vi "Encode DCW Parameters - 24ch.vi"(8 "ADD Parameters (in)":string, 9 "Scanner Settings":T2={"Scan1"=1, "Scan2"=1, "Scan3"=1, "Scan4"=1, "Scan5"=1, "Scan6"=1, "Scan7"=1, "Scan8"=1, "Scan9"=1, "Scan10"=1, "Scan11"=1, "Scan12"=1, "Scan13"=1, "Scan14"=1, "Scan15"=1, "Scan16"=1, "Scan17"=1, "Scan10 2"=1, "Scan11 2"=1, "Scan12 2"=1, "Scan13 2"=1, "Scan14 2"=1, "Scan15 2"=1, "Scan24"=1} {"Scan24" scale=0.0..2.0; "Scan15 2" scale=0.0..2.0; "Scan14 2" scale=0.0..2.0; "Scan13 2" scale=0.0..2.0; "Scan12 2" scale=0.0..2.0; "Scan11 2" scale=0.0..2.0; "Scan10 2" scale=0.0..2.0; "Scan17" scale=0.0..2.0; "Scan16" scale=0.0..2.0; "Scan15" scale=0.0..2.0; "Scan14" scale=0.0..2.0; "Scan13" scale=0.0..2.0; "Scan12" scale=0.0..2.0; "Scan11" scale=0.0..2.0; "Scan10" scale=0.0..2.0; "Scan9" scale=0.0..2.0; "Scan8" scale=0.0..2.0; "Scan7" scale=0.0..2.0; "Scan6" scale=0.0..2.0; "Scan5" scale=0.0..2.0; "Scan4" scale=0.0..2.0; "Scan3" min=0 max=2 scale=0.0..2.0; "Scan2" min=0 max=2 scale=0.0..2.0; "Scan1" min=0 max=2 scale=0.0..2.0}, 10 "Internal Scanner Exists?":bool, 11 "DCW Test Parameters out":T1={"Voltage (1500)"=1500, "High Limit(0.0 - 10,000 microamps) (10)"=10000.0, "Low Limit(0.0 - 10,000 microamps) (0)"=0.0, "Ramp Up Time (0.4 - 999.9 seconds) (0.4)"=0.4, "Dwell Time (0, 0.4 - 999.9 seconds) (1)"=1.0, "Ramp Down Time (0, 1.0 - 999.9 seconds) (0) "=0.0, "Charge LO (0.0 - 350uA)"=0.0, "Arc Sense (1 - 9) (5)"=5, "Arc Detect (F: Off)"=FALSE, "Continuity (F: Off)"=FALSE, "Auto Charge LO (F: Off)"=FALSE, "Low Range (F: Off)"=FALSE, "Offset (0.0 - 10,000uA)"=0.0, "Ramp-Hi (0.0 - 10,000uA)"=0.0, "Range (F: AUTO)"=enum."AUTO"} {"Ramp-Hi (0.0 - 10,000uA)" format="%.2f"; "Offset (0.0 - 10,000uA)" format="%.2f"; "Ramp Down Time (0, 1.0 - 999.9 seconds) (0)" format="%.1f"; "Charge LO (0.0 - 350uA)" format="%.2f"; "Dwell Time (0, 0.4 - 999.9 seconds) (1)" format="%.1f"; "Ramp Up Time (0.4 - 999.9 seconds) (0.4)" format="%.1f"; "Low Limit(0.0 - 10,000 microamps) (0)" format="%.1f"; "High Limit(0.0 - 10,000 microamps) (10)" format="%.1f"}) -> (0 "Scanner Settings":T2={"Scan1"=1, "Scan2"=1, "Scan3"=1, "Scan4"=1, "Scan5"=1, "Scan6"=1, "Scan7"=1, "Scan8"=1, "Scan9"=1, "Scan10"=1, "Scan11"=1, "Scan12"=1, "Scan13"=1, "Scan14"=1, "Scan15"=1, "Scan16"=1, "Scan17"=1, "Scan10 2"=1, "Scan11 2"=1, "Scan12 2"=1, "Scan13 2"=1, "Scan14 2"=1, "Scan15 2"=1, "Scan24"=1} {"Scan24" scale=0.0..2.0; "Scan15 2" scale=0.0..2.0; "Scan14 2" scale=0.0..2.0; "Scan13 2" scale=0.0..2.0; "Scan12 2" scale=0.0..2.0; "Scan11 2" scale=0.0..2.0; "Scan10 2" scale=0.0..2.0; "Scan17" scale=0.0..2.0; "Scan16" scale=0.0..2.0; "Scan15" scale=0.0..2.0; "Scan14" scale=0.0..2.0; "Scan13" scale=0.0..2.0; "Scan12" scale=0.0..2.0; "Scan11" scale=0.0..2.0; "Scan10" scale=0.0..2.0; "Scan9" scale=0.0..2.0; "Scan8" scale=0.0..2.0; "Scan7" scale=0.0..2.0; "Scan6" scale=0.0..2.0; "Scan5" scale=0.0..2.0; "Scan4" scale=0.0..2.0; "Scan3" min=0 max=2 scale=0.0..2.0; "Scan2" min=0 max=2 scale=0.0..2.0; "Scan1" min=0 max=2 scale=0.0..2.0}, 1 "DCW Test Parameters out":T1={"Voltage (1500)"=1500, "High Limit(0.0 - 10,000 microamps) (10)"=10000.0, "Low Limit(0.0 - 10,000 microamps) (0)"=0.0, "Ramp Up Time (0.4 - 999.9 seconds) (0.4)"=0.4, "Dwell Time (0, 0.4 - 999.9 seconds) (1)"=1.0, "Ramp Down Time (0, 1.0 - 999.9 seconds) (0) "=0.0, "Charge LO (0.0 - 350uA)"=0.0, "Arc Sense (1 - 9) (5)"=5, "Arc Detect (F: Off)"=FALSE, "Continuity (F: Off)"=FALSE, "Auto Charge LO (F: Off)"=FALSE, "Low Range (F: Off)"=FALSE, "Offset (0.0 - 10,000uA)"=0.0, "Ramp-Hi (0.0 - 10,000uA)"=0.0, "Range (F: AUTO)"=enum."AUTO"} {"Ramp-Hi (0.0 - 10,000uA)" format="%.2f"; "Offset (0.0 - 10,000uA)" format="%.2f"; "Ramp Down Time (0, 1.0 - 999.9 seconds) (0)" format="%.1f"; "Charge LO (0.0 - 350uA)" format="%.2f"; "Dwell Time (0, 0.4 - 999.9 seconds) (1)" format="%.1f"; "Ramp Up Time (0.4 - 999.9 seconds) (0.4)" format="%.1f"; "Low Limit(0.0 - 10,000 microamps) (0)" format="%.1f"; "High Limit(0.0 - 10,000 microamps) (10)" format="%.1f"}, 3 "Add Parameters":string)   [LabVIEW 2020, in "Associated Research 78XX Series.lvlib"]
uses:
  <instrlib>/Associated Research 78XX Series/Associated Research 78XX Series.lvlib
  <instrlib>/Associated Research 78XX Series/Public/Configure/Steps/Low Level/Scanner Settings - 24ch.ctl
  <instrlib>/Associated Research 78XX Series/Public/Configure/Steps/Low Level/DCW Test Parameters.ctl
panel:
  # "On\nOff"
  # "On\nOff"
  # "On\nOff"
  # "Fixed\nAuto"
  # "On\nOff"
  # "On\nOff"
  # "On\nOff"
  # "On\nOff"
  # "Fixed\nAuto"
  # "On\nOff"
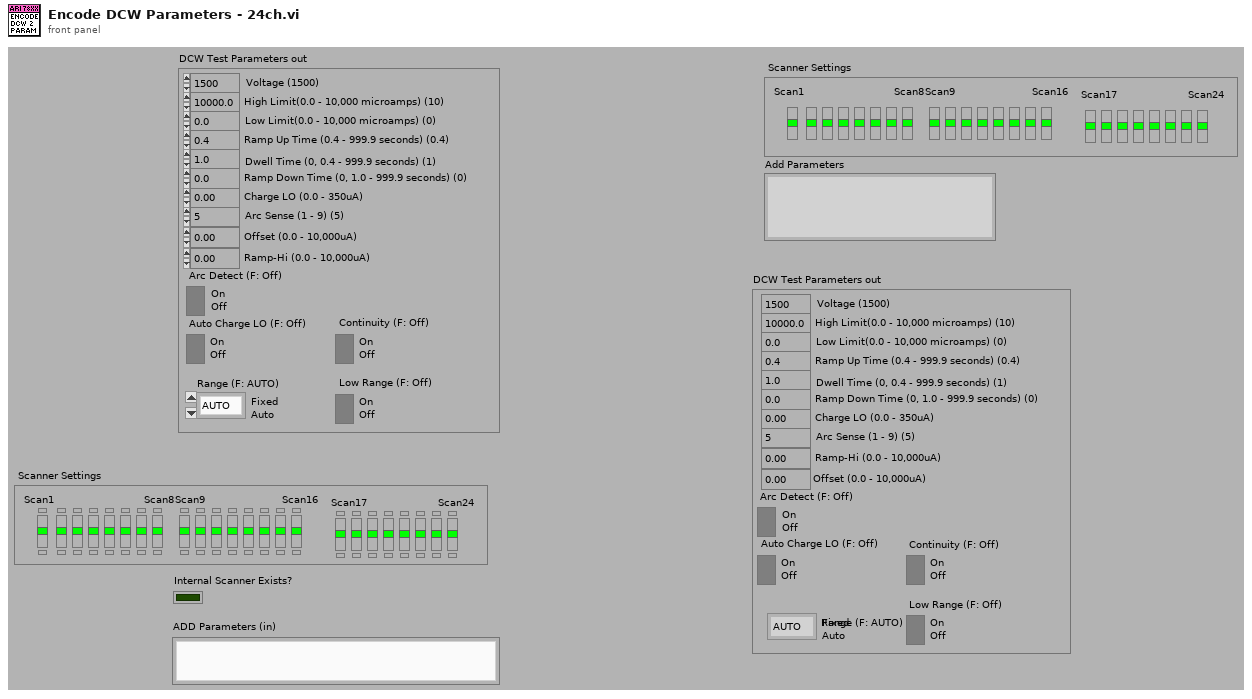
[diagram p1: front panel]
types:
  T1 = typedef "Associated Research 78XX Series.lvlib/DCW Test Parameters.ctl" = cluster{"Voltage (1500)":i32, "High Limit(0.0 - 10,000 microamps) (10)":dbl, "Low Limit(0.0 - 10,000 microamps) (0)":dbl, "Ramp Up Time (0.4 - 999.9 seconds) (0.4)":dbl, "Dwell Time (0, 0.4 - 999.9 seconds) (1)":dbl, "Ramp Down Time (0, 1.0 - 999.9 seconds) (0) ":dbl, "Charge LO (0.0 - 350uA)":dbl, "Arc Sense (1 - 9) (5)":i32, "Arc Detect (F: Off)":bool, "Continuity (F: Off)":bool, "Auto Charge LO (F: Off)":bool, "Low Range (F: Off)":bool, "Offset (0.0 - 10,000uA)":dbl, "Ramp-Hi (0.0 - 10,000uA)":dbl, "Range (F: AUTO)":enum16{"AUTO", "FIXED"}}
  T2 = typedef "Associated Research 78XX Series.lvlib/Scanner Settings - 24ch.ctl" = cluster{"Scan1":i32, "Scan2":i32, "Scan3":i32, "Scan4":i32, "Scan5":i32, "Scan6":i32, "Scan7":i32, "Scan8":i32, "Scan9":i32, "Scan10":i32, "Scan11":i32, "Scan12":i32, "Scan13":i32, "Scan14":i32, "Scan15":i32, "Scan16":i32, "Scan17":i32, "Scan10 2":i32, "Scan11 2":i32, "Scan12 2":i32, "Scan13 2":i32, "Scan14 2":i32, "Scan15 2":i32, "Scan24":i32}
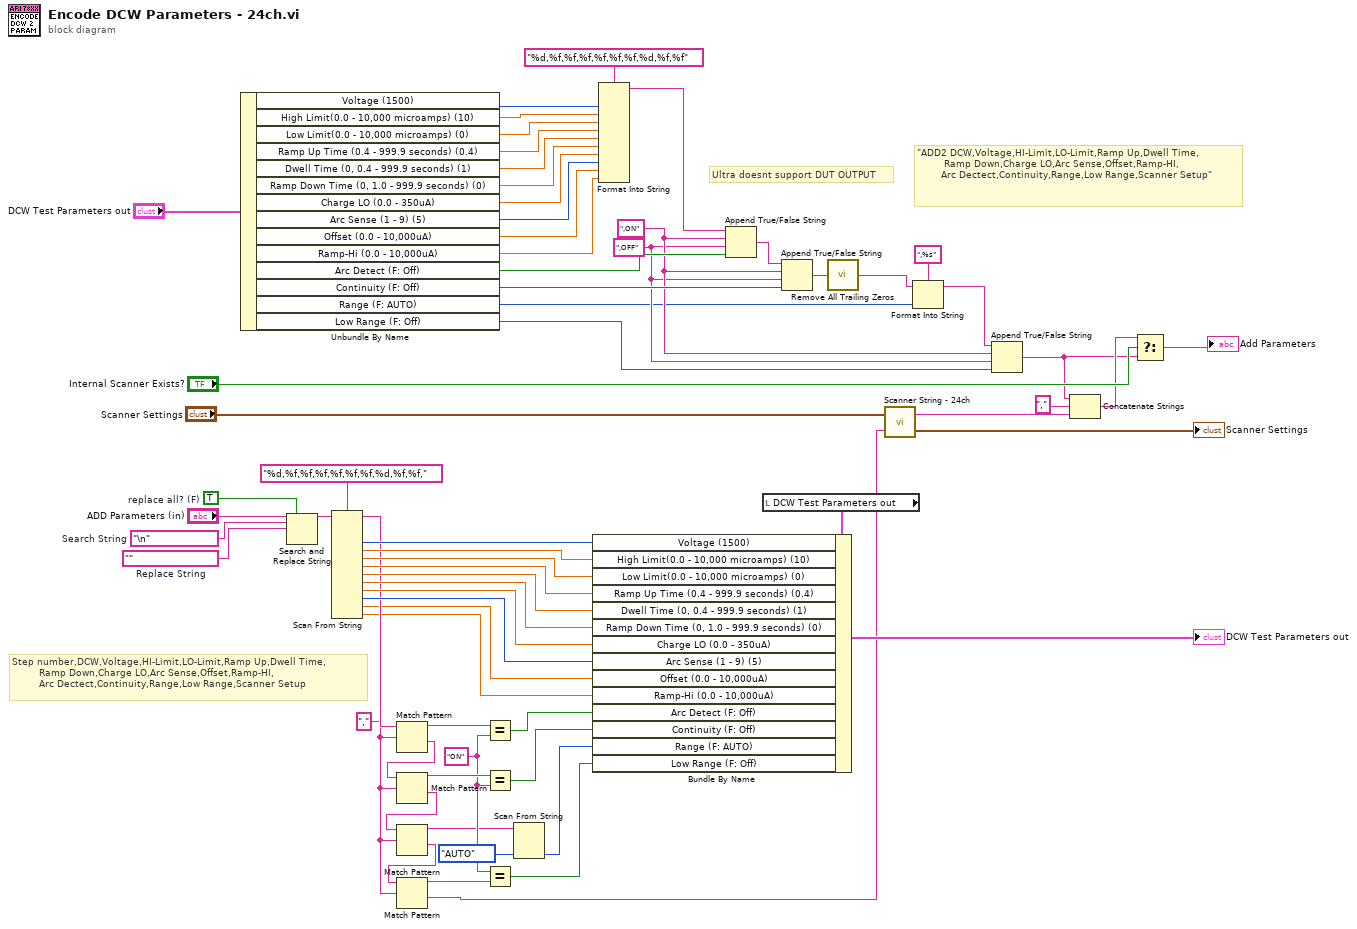
[diagram p0: block diagram]
diagram:
  w28 = TRUE  # replace all? (F)
  w29 = ""  # Replace String
  w30 = "\n"  # Search String
  w31 = "ON" ("y")
  w33 = "," ("regular expression")
  w19 = ",OFF" ("false string")
  w20 = ",ON" ("true string")
  # "Step number,DCW,Voltage,HI-Limit,LO-Limit,Ramp Up,Dwell Time,\n         Ramp Down,Charge LO,Arc Sense,Offset,Ramp-HI, \n         Arc Dectect,Continuity,Range,Low Range,Scanner Setup"
  # "\"ADD2 DCW,Voltage,HI-Limit,LO-Limit,Ramp Up,Dwell Time,\n         Ramp Down,Charge LO,Arc Sense,Offset,Ramp-HI,\n        Arc Dectect,Continuity,Range,Low Range,Scanner Setup\""
  # "Ultra doesnt support DUT OUTPUT"
  n1 = Unbundle By Name("DCW Test Parameters out") -> ("Voltage (1500)"=w66:i32, "High Limit(0.0 - 10,000 microamps) (10)"=w11:dbl, "Low Limit(0.0 - 10,000 microamps) (0)"=w65:dbl, "Ramp Up Time (0.4 - 999.9 seconds) (0.4)"=w64:dbl, "Dwell Time (0, 0.4 - 999.9 seconds) (1)"=w63:dbl, "Ramp Down Time (0, 1.0 - 999.9 seconds) (0)"=w62:dbl, "Charge LO (0.0 - 350uA)"=w61:dbl, "Arc Sense (1 - 9) (5)"=w60:i32, "Offset (0.0 - 10,000uA)"=w22:dbl, "Ramp-Hi (0.0 - 10,000uA)"=w13:dbl, "Arc Detect (F: Off)"=w54:bool, "Continuity (F: Off)"=w53:bool, "Range (F: AUTO)"=w5:enum16{"AUTO", "FIXED"}, "Low Range (F: Off)"=w18:bool)
  n2 = Search and Replace String(replace all?=w28, input string="ADD Parameters (in)", search string=w30, replace string=w29) -> (result string=w26:string)  [unwired: 4 in, 3 out]
  n3 = Scan From String(format string="%d,%f,%f,%f,%f,%f,%f,%d,%f,%f," ("Format String"), input string=w26) -> (remaining string=w41:string, output 1=w49:i32, output 2=w48:dbl, output 3=w47:dbl, output 4=w46:dbl, output 5=w45:dbl, output 6=w44:dbl, output 7=w43:dbl, output 8=w42:i32, output 9=w21:dbl, output 10=w16:dbl)  [unwired: 12 in, 2 out]
  n4 = Match Pattern(string=w41, regular expression=w33) -> (before substring=w38:string, after substring=w40:string)  [unwired: 1 in, 2 out]
  n5 = Match Pattern(string=w40, regular expression=w33) -> (before substring=w36:string, after substring=w39:string)  [unwired: 1 in, 2 out]
  n6 = Match Pattern(string=w39, regular expression=w33) -> (before substring=w15:string, after substring=w25:string)  [unwired: 1 in, 2 out]
  n7 = Match Pattern(string=w25, regular expression=w33) -> (before substring=w32:string, after substring=w2:string)  [unwired: 1 in, 2 out]
  n8 = Equal?(x=w38, y=w31) -> (x = y?=w37:bool)
  n9 = Equal?(x=w36, y=w31) -> (x = y?=w35:bool)
  n10 = Equal?(x=w31, y=w32) -> (x = y?=w23:bool)
  n11 = Scan From String(input string=w15, default 1=enum16{"AUTO", "FIXED"}."AUTO") -> (output 1=w14:enum16{"AUTO", "FIXED"})  [unwired: 3 in, 3 out]
  n12 = Format Into String(format string="%d,%f,%f,%f,%f,%f,%f,%d,%f,%f" ("Format String"), w66, w11, w65, w64, w63, w62, w61, w60, w22, w13) -> (resulting string=w12:string)  [unwired: 2 in, 1 out]
  n13 = Append True/False String(1:w54, 2:w19, 3:w20, 4:w12) -> (0:w59:string)
  n14 = local read "DCW Test Parameters out"() -> (w24:T1)
  n15 = Bundle By Name(cluster=w24, "Voltage (1500)"=w49, "High Limit(0.0 - 10,000 microamps) (10)"=w48, "Low Limit(0.0 - 10,000 microamps) (0)"=w47, "Ramp Up Time (0.4 - 999.9 seconds) (0.4)"=w46, "Dwell Time (0, 0.4 - 999.9 seconds) (1)"=w45, "Ramp Down Time (0, 1.0 - 999.9 seconds) (0)"=w44, "Charge LO (0.0 - 350uA)"=w43, "Arc Sense (1 - 9) (5)"=w42, "Offset (0.0 - 10,000uA)"=w21, "Ramp-Hi (0.0 - 10,000uA)"=w16, "Arc Detect (F: Off)"=w37, "Continuity (F: Off)"=w35, "Range (F: AUTO)"=w14, "Low Range (F: Off)"=w23) -> (→"DCW Test Parameters out":T1)
  n16 = Append True/False String(1:w53, 2:w19, 3:w20, 4:w59) -> (0:w57:string)
  n17 = call <instrlib>:"Remove All Trailing Zeros.vi"("String in"=w57) -> ("String out"=w3:string)
  n18 = call <instrlib>:"Scanner String - 24ch.vi"("Scanner String (in)"=w2, "Scanner Settings"="Scanner Settings") -> ("Scanner Settings"=→"Scanner Settings":T2, "Scanner String (out)"=w56:string)
  n19 = Format Into String(format string=",%s", initial string=w3, w5) -> (resulting string=w4:string)  [unwired: 1 in, 1 out]
  n20 = Append True/False String(1:w18, 2:w19, 3:w20, 4:w4) -> (0:w17:string)
  n21 = Concatenate Strings(w17, "," ("Substring"), w56) -> (w34:string)
  n22 = Select(t=w34, s="Internal Scanner Exists?", f=w17) -> (s? t:f=→"Add Parameters":string)
